vi "FeedbackDecode_BuildMSMSMvnt.vi"(4 "CompArray":T2(array[cluster])=[{"Name"="\"LittleSphereJ\"", "Type"="\"Trans3Joint\"", "ID"="J", "Num"="86", "COM"=[], "Offset"=[], "RotationAxis"=[], "OrientationMatrix"=[[1.0, 0.0, 0.0], [0.0, 1.0, 0.0], [0.0, 0.0, 1.0]], "MinAngle"=nan, "MaxAngle"=nan, "InboardID"="S", "InboardNum"="1110", "InboardCOM"=[0.0, 0.0, 0.0], "OutboardID"="S", "OutboardNum"="84", "OutboardCOM"=[0.0, 0.0, 0.0]}, {"Name"="\"IndexSphereJ\"", "Type"="\"Trans3Joint\"", "ID"="J", "Num"="94", "COM"=[], "Offset"=[], "RotationAxis"=[], "OrientationMatrix"=[[1.0, 0.0, 0.0], [0.0, 1.0, 0.0], [0.0, 0.0, 1.0]], "MinAngle"=nan, "MaxAngle"=nan, "InboardID"="S", "InboardNum"="1110", "InboardCOM"=[0.0, 0.0, 0.0], "OutboardID"="S", "OutboardNum"="92", "OutboardCOM"=[0.0, 0.0, 0.0]}, {"Name"="\"LittleKnuckle\"", "Type"="\"PinJoint\"", "ID"="J", "Num"="1160", "COM"=[], "Offset"=[], "RotationAxis"=[-0.982409, 0.0686967, 0.173648], "OrientationMatrix"=[[1.0, 0.0, 0.0], [0.0, 1.0, 0.0], [0.0, 0.0, 1.0]], "MinAngle"=0.0, "MaxAngle"=3.140021857262998, "InboardID"="S", "InboardNum"="1122", "InboardCOM"=[-0.01026417, -0.01431899999999997, 0.005183300000000002], "OutboardID"="S", "OutboardNum"="112", "OutboardCOM"=[0.0, 0.0, 0.0]}, {"Name"="\"LittleSide\"", "Type"="\"PinJoint\"", "ID"="J", "Num"="1161", "COM"=[], "Offset"=[], "RotationAxis"=[0.173225, -0.0121131, -0.984808], "OrientationMatrix"=[[1.0, 0.0, 0.0], [0.0, 1.0, 0.0], [0.0, 0.0, 1.0]], "MinAngle"=0.0, "MaxAngle"=3.140021857262998, "InboardID"="S", "InboardNum"="1110", "InboardCOM"=[-0.02813713, -0.080592, -0.0049779], "OutboardID"="S", "OutboardNum"="1122", "OutboardCOM"=[0.0, 0.0, 0.0]}, {"Name"="\"RingPIP\"", "Type"="\"PinJoint\"", "ID"="J", "Num"="1162", "COM"=[], "Offset"=[], "RotationAxis"=[-0.993768, 0.069491, 0.0871557], "OrientationMatrix"=[[1.0, 0.0, 0.0], [0.0, 1.0, 0.0], [0.0, 0.0, 1.0]], "MinAngle"=0.0, "MaxAngle"=3.140021857262998, "InboardID"="S", "InboardNum"="1125", "InboardCOM"=[-0.00263497, -0.03339700000000001, 2.619999999999706e-05], "OutboardID"="S", "OutboardNum"="1121", "OutboardCOM"=[0.0, 0.0, 0.0]}, {"Name"="\"ThumbKnuckle\"", "Type"="\"PinJoint\"", "ID"="J", "Num"="1163", "COM"=[], "Offset"=[], "RotationAxis"=[-0.130028, -0.197163, -0.97171], "OrientationMatrix"=[[1.0, 0.0, 0.0], [0.0, 1.0, 0.0], [0.0, 0.0, 1.0]], "MinAngle"=0.0, "MaxAngle"=3.140021857262998, "InboardID"="S", "InboardNum"="1113", "InboardCOM"=[0.0221366, -0.0038129999999999553, 0.00214783], "OutboardID"="S", "OutboardNum"="111", "OutboardCOM"=[0.0, 0.0, 0.0]}, {"Name"="\"RingSide\"", "Type"="\"PinJoint\"", "ID"="J", "Num"="1164", "COM"=[], "Offset"=[], "RotationAxis"=[0.0869434, -0.00607968, -0.996195], "OrientationMatrix"=[[1.0, 0.0, 0.0], [0.0, 1.0, 0.0], [0.0, 0.0, 1.0]], "MinAngle"=0.0, "MaxAngle"=3.140021857262998, "InboardID"="S", "InboardNum"="1110", "InboardCOM"=[-0.0087988, -0.08356699999999995, -0.008058199999999998], "OutboardID"="S", "OutboardNum"="1123", "OutboardCOM"=[0.0, 0.0, 0.0]}, {"Name"="\"RingKnuckle\"", "Type"="\"PinJoint\"", "ID"="J", "Num"="1165", "COM"=[], "Offset"=[], "RotationAxis"=[-0.993768, 0.069491, 0.0871557], "OrientationMatrix"=[[1.0, 0.0, 0.0], [0.0, 1.0, 0.0], [0.0, 0.0, 1.0]], "MinAngle"=0.0, "MaxAngle"=3.140021857262998, "InboardID"="S", "InboardNum"="1123", "InboardCOM"=[-0.01067969, -0.014290000000000025, 0.0043582], "OutboardID"="S", "OutboardNum"="1125", "OutboardCOM"=[0.0, 0.0, 0.0]}, {"Name"="\"ShoulderRoll\"", "Type"="\"PinJoint\"", "ID"="J", "Num"="1166", "COM"=[], "Offset"=[], "RotationAxis"=[0.0, -1.0, 0.0], "OrientationMatrix"=[[1.0, 0.0, 0.0], [0.0, 1.0, 0.0], [0.0, 0.0, 1.0]], "MinAngle"=0.0, "MaxAngle"=3.140021857262998, "InboardID"="S", "InboardNum"="1127", "InboardCOM"=[0.0346, -0.26093099999999997, 0.0], "OutboardID"="S", "OutboardNum"="116", "OutboardCOM"=[0.0, 0.0, 0.0]}, {"Name"="\"MiddleDIP\"", "Type"="\"PinJoint\"", "ID"="J", "Num"="1167", "COM"=[], "Offset"=[], "RotationAxis"=[-1.0, 0.0, 0.0], "OrientationMatrix"=[[1.0, 0.0, 0.0], [0.0, 1.0, 0.0], [0.0, 0.0, 1.0]], "MinAngle"=0.0, "MaxAngle"=3.14, "InboardID"="S", "InboardNum"="113", "InboardCOM"=[0.0197, -0.022077000000000013, -0.0010000000000000009], "OutboardID"="S", "OutboardNum"="1114", "OutboardCOM"=[0.0, 0.0, 0.0]}, {"Name"="\"IndexDIP\"", "Type"="\"PinJoint\"", "ID"="J", "Num"="1168", "COM"=[], "Offset"=[], "RotationAxis"=[-1.0, 0.0, 0.0], "OrientationMatrix"=[[1.0, 0.0, 0.0], [0.0, 1.0, 0.0], [0.0, 0.0, 1.0]], "MinAngle"=0.0, "MaxAngle"=3.140021857262998, "InboardID"="S", "InboardNum"="1124", "InboardCOM"=[0.019699999999999995, -0.017971999999999988, -0.0009999999999999974], "OutboardID"="S", "OutboardNum"="1117", "OutboardCOM"=[0.0, 0.0, 0.0]}, {"Name"="\"IndexKnuckle\"", "Type"="\"PinJoint\"", "ID"="J", "Num"="1169", "COM"=[], "Offset"=[], "RotationAxis"=[-1.0, 0.0, 0.0], "OrientationMatrix"=[[1.0, 0.0, 0.0], [0.0, 1.0, 0.0], [0.0, 0.0, 1.0]], "MinAngle"=0.0, "MaxAngle"=3.140021857262998, "InboardID"="S", "InboardNum"="1118", "InboardCOM"=[-0.0071716, -0.017827999999999955, 0.0025407999999999993], "OutboardID"="S", "OutboardNum"="1126", "OutboardCOM"=[0.0, 0.0, 0.0]}, {"Name"="\"MiddleKnuckle\"", "Type"="\"PinJoint\"", "ID"="J", "Num"="1170", "COM"=[], "Offset"=[], "RotationAxis"=[-1.0, 0.0, 0.0], "OrientationMatrix"=[[1.0, 0.0, 0.0], [0.0, 1.0, 0.0], [0.0, 0.0, 1.0]], "MinAngle"=0.0, "MaxAngle"=3.140021857262998, "InboardID"="S", "InboardNum"="1110", "InboardCOM"=[-0.00031180000000000097, -0.09855000000000003, -0.0048641], "OutboardID"="S", "OutboardNum"="1119", "OutboardCOM"=[0.0, 0.0, 0.0]}, {"Name"="\"RingSphereJ\"", "Type"="\"Trans3Joint\"", "ID"="J", "Num"="15", "COM"=[], "Offset"=[], "RotationAxis"=[], "OrientationMatrix"=[[1.0, 0.0, 0.0], [0.0, 1.0, 0.0], [0.0, 0.0, 1.0]], "MinAngle"=nan, "MaxAngle"=nan, "InboardID"="S", "InboardNum"="1110", "InboardCOM"=[0.0, 0.0, 0.0], "OutboardID"="S", "OutboardNum"="18", "OutboardCOM"=[0.0, 0.0, 0.0]}, {"Name"="\"MiddleSphereJ\"", "Type"="\"Trans3Joint\"", "ID"="J", "Num"="11", "COM"=[], "Offset"=[], "RotationAxis"=[], "OrientationMatrix"=[[1.0, 0.0, 0.0], [0.0, 1.0, 0.0], [0.0, 0.0, 1.0]], "MinAngle"=nan, "MaxAngle"=nan, "InboardID"="S", "InboardNum"="1110", "InboardCOM"=[0.0, 0.0, 0.0], "OutboardID"="S", "OutboardNum"="14", "OutboardCOM"=[0.0, 0.0, 0.0]}, {"Name"="\"ThumbSphereJ\"", "Type"="\"Trans3Joint\"", "ID"="J", "Num"="23", "COM"=[], "Offset"=[], "RotationAxis"=[], "OrientationMatrix"=[[1.0, 0.0, 0.0], [0.0, 1.0, 0.0], [0.0, 0.0, 1.0]], "MinAngle"=nan, "MaxAngle"=nan, "InboardID"="S", "InboardNum"="1110", "InboardCOM"=[0.0, 0.0, 0.0], "OutboardID"="S", "OutboardNum"="22", "OutboardCOM"=[0.0, 0.0, 0.0]}, {"Name"="\"RingDIP\"", "Type"="\"PinJoint\"", "ID"="J", "Num"="1144", "COM"=[], "Offset"=[], "RotationAxis"=[-0.993768, 0.069491, 0.0871557], "OrientationMatrix"=[[1.0, 0.0, 0.0], [0.0, 1.0, 0.0], [0.0, 0.0, 1.0]], "MinAngle"=0.0, "MaxAngle"=3.140021857262998, "InboardID"="S", "InboardNum"="1121", "InboardCOM"=[0.01818386, -0.020046000000000008, -0.002713199999999999], "OutboardID"="S", "OutboardNum"="115", "OutboardCOM"=[0.0, 0.0, 0.0]}, {"Name"="\"ElbowPitch\"", "Type"="\"PinJoint\"", "ID"="J", "Num"="1145", "COM"=[], "Offset"=[], "RotationAxis"=[0.0, 0.0, 1.0], "OrientationMatrix"=[[1.0, 0.0, 0.0], [0.0, 1.0, 0.0], [0.0, 0.0, 1.0]], "MinAngle"=0.0, "MaxAngle"=3.140021857262998, "InboardID"="S", "InboardNum"="116", "InboardCOM"=[0.019, -0.013836000000000015, -0.009000000000000001], "OutboardID"="S", "OutboardNum"="1111", "OutboardCOM"=[0.0, 0.0, 0.0]}, {"Name"="\"WristPitch\"", "Type"="\"PinJoint\"", "ID"="J", "Num"="1146", "COM"=[], "Offset"=[], "RotationAxis"=[-1.0, 0.0, 0.0], "OrientationMatrix"=[[1.0, 0.0, 0.0], [0.0, 1.0, 0.0], [0.0, 0.0, 1.0]], "MinAngle"=-0.7853981633974483, "MaxAngle"=0.7853981633974483, "InboardID"="S", "InboardNum"="114", "InboardCOM"=[0.042499999999999996, -0.16914000000000007, 0.0], "OutboardID"="S", "OutboardNum"="119", "OutboardCOM"=[0.0, 0.0, 0.0]}, {"Name"="\"ThumbDIP\"", "Type"="\"PinJoint\"", "ID"="J", "Num"="1147", "COM"=[], "Offset"=[], "RotationAxis"=[-0.130028, -0.197163, -0.97171], "OrientationMatrix"=[[1.0, 0.0, 0.0], [0.0, 1.0, 0.0], [0.0, 0.0, 1.0]], "MinAngle"=0.0, "MaxAngle"=3.14, "InboardID"="S", "InboardNum"="111", "InboardCOM"=[0.018637, -0.022448000000000023, -0.01061123], "OutboardID"="S", "OutboardNum"="1116", "OutboardCOM"=[0.0, 0.0, 0.0]}, {"Name"="\"IndexSide\"", "Type"="\"PinJoint\"", "ID"="J", "Num"="1148", "COM"=[], "Offset"=[], "RotationAxis"=[0.0, 0.0, -1.0], "OrientationMatrix"=[[1.0, 0.0, 0.0], [0.0, 1.0, 0.0], [0.0, 0.0, 1.0]], "MinAngle"=0.0, "MaxAngle"=3.140021857262998, "InboardID"="S", "InboardNum"="1110", "InboardCOM"=[0.027229700000000003, -0.07779400000000003, -0.0051141], "OutboardID"="S", "OutboardNum"="1118", "OutboardCOM"=[0.0, 0.0, 0.0]}, {"Name"="\"MiddlePIP\"", "Type"="\"PinJoint\"", "ID"="J", "Num"="1149", "COM"=[], "Offset"=[], "RotationAxis"=[-1.0, 0.0, 0.0], "OrientationMatrix"=[[1.0, 0.0, 0.0], [0.0, 1.0, 0.0], [0.0, 0.0, 1.0]], "MinAngle"=0.0, "MaxAngle"=3.140021857262998, "InboardID"="S", "InboardNum"="1119", "InboardCOM"=[-0.0002999999999999982, -0.0383, 0.0], "OutboardID"="S", "OutboardNum"="113", "OutboardCOM"=[0.0, 0.0, 0.0]}, {"Name"="\"ShoulderYaw\"", "Type"="\"PinJoint\"", "ID"="J", "Num"="1150", "COM"=[], "Offset"=[], "RotationAxis"=[0.0, 0.0, 1.0], "OrientationMatrix"=[[1.0, 0.0, 0.0], [0.0, 1.0, 0.0], [0.0, 0.0, 1.0]], "MinAngle"=0.0, "MaxAngle"=3.140021857262998, "InboardID"="S", "InboardNum"="117", "InboardCOM"=[-1.45121e-10, 0.000384746, -0.003098433], "OutboardID"="S", "OutboardNum"="1120", "OutboardCOM"=[0.0, 0.0, 0.0]}, {"Name"="\"ThumbSide\"", "Type"="\"PinJoint\"", "ID"="J", "Num"="1151", "COM"=[], "Offset"=[], "RotationAxis"=[0.691978, 0.683845, -0.23135], "OrientationMatrix"=[[1.0, 0.0, 0.0], [0.0, 1.0, 0.0], [0.0, 0.0, 1.0]], "MinAngle"=-0.7853981633974483, "MaxAngle"=0.7853981633974483, "InboardID"="S", "InboardNum"="118", "InboardCOM"=[0.008416800000000002, -0.028861000000000026, 0.0017169000000000004], "OutboardID"="S", "OutboardNum"="1113", "OutboardCOM"=[0.0, 0.0, 0.0]}, {"Name"="\"LittleDIP\"", "Type"="\"PinJoint\"", "ID"="J", "Num"="1152", "COM"=[], "Offset"=[], "RotationAxis"=[-0.982409, 0.0686967, 0.173648], "OrientationMatrix"=[[1.0, 0.0, 0.0], [0.0, 1.0, 0.0], [0.0, 0.0, 1.0]], "MinAngle"=0.0, "MaxAngle"=3.140021857262998, "InboardID"="S", "InboardNum"="1115", "InboardCOM"=[0.01887955, -0.014112000000000013, -0.004509900000000001], "OutboardID"="S", "OutboardNum"="1112", "OutboardCOM"=[0.0, 0.0, 0.0]}, {"Name"="\"WristYaw\"", "Type"="\"PinJoint\"", "ID"="J", "Num"="1153", "COM"=[], "Offset"=[], "RotationAxis"=[0.0, 0.0, -1.0], "OrientationMatrix"=[[1.0, 0.0, 0.0], [0.0, 1.0, 0.0], [0.0, 0.0, 1.0]], "MinAngle"=-0.7853981633974483, "MaxAngle"=0.7853981633974483, "InboardID"="S", "InboardNum"="119", "InboardCOM"=[-0.0425218, -0.006901999999999964, -0.004796100000000001], "OutboardID"="S", "OutboardNum"="1110", "OutboardCOM"=[0.0, 0.0, 0.0]}, {"Name"="\"IndexPIP\"", "Type"="\"PinJoint\"", "ID"="J", "Num"="1154", "COM"=[], "Offset"=[], "RotationAxis"=[-1.0, 0.0, 0.0], "OrientationMatrix"=[[1.0, 0.0, 0.0], [0.0, 1.0, 0.0], [0.0, 0.0, 1.0]], "MinAngle"=0.0, "MaxAngle"=3.140021857262998, "InboardID"="S", "InboardNum"="1126", "InboardCOM"=[-0.00030000000000000165, -0.03400000000000003, 0.0], "OutboardID"="S", "OutboardNum"="1124", "OutboardCOM"=[0.0, 0.0, 0.0]}, {"Name"="\"LittlePIP\"", "Type"="\"PinJoint\"", "ID"="J", "Num"="1155", "COM"=[], "Offset"=[], "RotationAxis"=[-0.982409, 0.0686967, 0.173648], "OrientationMatrix"=[[1.0, 0.0, 0.0], [0.0, 1.0, 0.0], [0.0, 0.0, 1.0]], "MinAngle"=0.0, "MaxAngle"=3.140021857262998, "InboardID"="S", "InboardNum"="112", "InboardCOM"=[-0.0021084, -0.02591600000000005, 5.209999999999937e-05], "OutboardID"="S", "OutboardNum"="1115", "OutboardCOM"=[0.0, 0.0, 0.0]}, {"Name"="\"ThumbMeta\"", "Type"="\"PinJoint\"", "ID"="J", "Num"="1156", "COM"=[], "Offset"=[], "RotationAxis"=[-0.0212682, -0.997909, -0.0610298], "OrientationMatrix"=[[1.0, 0.0, 0.0], [0.0, 1.0, 0.0], [0.0, 0.0, 1.0]], "MinAngle"=0.0, "MaxAngle"=3.14, "InboardID"="S", "InboardNum"="1110", "InboardCOM"=[0.015011799999999999, -0.011859999999999982, 0.0126182], "OutboardID"="S", "OutboardNum"="118", "OutboardCOM"=[0.0, 0.0, 0.0]}, {"Name"="\"ShoulderOblique\"", "Type"="\"PinJoint\"", "ID"="J", "Num"="1157", "COM"=[], "Offset"=[], "RotationAxis"=[0.57735, 0.57735, 0.57735], "OrientationMatrix"=[[1.0, 0.0, 0.0], [0.0, 1.0, 0.0], [0.0, 0.0, 1.0]], "MinAngle"=0.0, "MaxAngle"=3.14, "InboardID"="S", "InboardNum"="12", "InboardCOM"=[-0.09, -0.05, -0.26], "OutboardID"="S", "OutboardNum"="117", "OutboardCOM"=[0.0, 0.0, 0.0]}, {"Name"="\"ShoulderPitch\"", "Type"="\"PinJoint\"", "ID"="J", "Num"="1158", "COM"=[], "Offset"=[], "RotationAxis"=[-1.0, 0.0, 0.0], "OrientationMatrix"=[[1.0, 0.0, 0.0], [0.0, 1.0, 0.0], [0.0, 0.0, 1.0]], "MinAngle"=0.0, "MaxAngle"=3.140021857262998, "InboardID"="S", "InboardNum"="1120", "InboardCOM"=[-0.0346, -0.005, -0.0125], "OutboardID"="S", "OutboardNum"="1127", "OutboardCOM"=[0.0, 0.0, 0.0]}, {"Name"="\"WristRoll\"", "Type"="\"PinJoint\"", "ID"="J", "Num"="1159", "COM"=[], "Offset"=[], "RotationAxis"=[0.0, -1.0, 0.0], "OrientationMatrix"=[[1.0, 0.0, 0.0], [0.0, 1.0, 0.0], [0.0, 0.0, 1.0]], "MinAngle"=-1.5707963267948966, "MaxAngle"=1.5707963267948966, "InboardID"="S", "InboardNum"="1111", "InboardCOM"=[0.0, -0.06298999999999999, 0.003020000000000002], "OutboardID"="S", "OutboardNum"="114", "OutboardCOM"=[0.0, 0.0, 0.0]}, {"Name"="\"WristSphereJ\"", "Type"="\"Trans3Joint\"", "ID"="J", "Num"="88", "COM"=[], "Offset"=[], "RotationAxis"=[], "OrientationMatrix"=[[1.0, 0.0, 0.0], [0.0, 1.0, 0.0], [0.0, 0.0, 1.0]], "MinAngle"=nan, "MaxAngle"=nan, "InboardID"="S", "InboardNum"="114", "InboardCOM"=[0.0, 0.0, 0.0], "OutboardID"="S", "OutboardNum"="87", "OutboardCOM"=[0.0, 0.0, 0.0]}, {"Name"="\"LittleSphere\"", "Type"="\"Segment\"", "ID"="S", "Num"="84", "COM"=[0.0, 0.0, 0.0], "Offset"=[0.0, 0.0, 0.0], "RotationAxis"=[], "OrientationMatrix"=[], "MinAngle"=nan, "MaxAngle"=nan, "InboardID"="", "InboardNum"="", "InboardCOM"=[], "OutboardID"="", "OutboardNum"="", "OutboardCOM"=[]}, {"Name"="\"IndexSphere\"", "Type"="\"Segment\"", "ID"="S", "Num"="92", "COM"=[0.0, 0.0, 0.0], "Offset"=[0.0, 0.0, 0.0], "RotationAxis"=[], "OrientationMatrix"=[], "MinAngle"=nan, "MaxAngle"=nan, "InboardID"="", "InboardNum"="", "InboardCOM"=[], "OutboardID"="", "OutboardNum"="", "OutboardCOM"=[]}, {"Name"="\"ShoulderHR\"", "Type"="\"Segment\"", "ID"="S", "Num"="1127", "COM"=[0.03942751, -0.096221, -2.3999999999996247e-06], "Offset"=[0.0346, 0.005, 0.01541], "RotationAxis"=[], "OrientationMatrix"=[], "MinAngle"=nan, "MaxAngle"=nan, "InboardID"="", "InboardNum"="", "InboardCOM"=[], "OutboardID"="", "OutboardNum"="", "OutboardCOM"=[]}, {"Name"="\"ThumbProximal\"", "Type"="\"Segment\"", "ID"="S", "Num"="111", "COM"=[0.010053400000000004, -0.01129800000000003, -0.003517029999999999], "Offset"=[-0.0645434, 0.563333, 0.00970317], "RotationAxis"=[], "OrientationMatrix"=[], "MinAngle"=nan, "MaxAngle"=nan, "InboardID"="", "InboardNum"="", "InboardCOM"=[], "OutboardID"="", "OutboardNum"="", "OutboardCOM"=[]}, {"Name"="\"LittleProximal\"", "Type"="\"Segment\"", "ID"="S", "Num"="112", "COM"=[0.0086144, -0.013174000000000019, -0.0019825000000000016], "Offset"=[0.0194231, 0.61371, 0.0259807], "RotationAxis"=[], "OrientationMatrix"=[], "MinAngle"=nan, "MaxAngle"=nan, "InboardID"="", "InboardNum"="", "InboardCOM"=[], "OutboardID"="", "OutboardNum"="", "OutboardCOM"=[]}, {"Name"="\"MiddleMedial\"", "Type"="\"Segment\"", "ID"="S", "Num"="113", "COM"=[0.009050299999999997, -0.011116000000000015, -0.0009771999999999975], "Offset"=[-0.0183664, 0.655649, 0.0310502], "RotationAxis"=[], "OrientationMatrix"=[], "MinAngle"=nan, "MaxAngle"=nan, "InboardID"="", "InboardNum"="", "InboardCOM"=[], "OutboardID"="", "OutboardNum"="", "OutboardCOM"=[]}, {"Name"="\"Forearm\"", "Type"="\"Segment\"", "ID"="S", "Num"="114", "COM"=[-1.860000000000056e-05, -0.08232500000000004, -9.750000000000036e-05], "Offset"=[-0.019, 0.342757, 0.02139], "RotationAxis"=[], "OrientationMatrix"=[], "MinAngle"=nan, "MaxAngle"=nan, "InboardID"="", "InboardNum"="", "InboardCOM"=[], "OutboardID"="", "OutboardNum"="", "OutboardCOM"=[]}, {"Name"="\"RingDistal\"", "Type"="\"Segment\"", "ID"="S", "Num"="115", "COM"=[-0.01039068, -0.008301000000000003, 0.0005073999999999981], "Offset"=[-0.0150486, 0.670099, 0.0325731], "RotationAxis"=[], "OrientationMatrix"=[], "MinAngle"=nan, "MaxAngle"=nan, "InboardID"="", "InboardNum"="", "InboardCOM"=[], "OutboardID"="", "OutboardNum"="", "OutboardCOM"=[]}, {"Name"="\"HR TO ELBOW_1\"", "Type"="\"Segment\"", "ID"="S", "Num"="116", "COM"=[0.0103972, 0.026906999999999986, 0.0011380000000000001], "Offset"=[0.0, 0.265931, 0.01541], "RotationAxis"=[], "OrientationMatrix"=[], "MinAngle"=nan, "MaxAngle"=nan, "InboardID"="", "InboardNum"="", "InboardCOM"=[], "OutboardID"="", "OutboardNum"="", "OutboardCOM"=[]}, {"Name"="\"ShoulderSocket\"", "Type"="\"Segment\"", "ID"="S", "Num"="117", "COM"=[0.0, 0.0, 0.0], "Offset"=[-1.45121e-10, 0.000384746, -0.000188433], "RotationAxis"=[], "OrientationMatrix"=[], "MinAngle"=nan, "MaxAngle"=nan, "InboardID"="", "InboardNum"="", "InboardCOM"=[], "OutboardID"="", "OutboardNum"="", "OutboardCOM"=[]}, {"Name"="\"ThumbRoll\"", "Type"="\"Segment\"", "ID"="S", "Num"="118", "COM"=[0.005574799999999998, -0.01721499999999998, -0.0012329999999999997], "Offset"=[-0.03399, 0.530659, 0.0135679], "RotationAxis"=[], "OrientationMatrix"=[], "MinAngle"=nan, "MaxAngle"=nan, "InboardID"="", "InboardNum"="", "InboardCOM"=[], "OutboardID"="", "OutboardNum"="", "OutboardCOM"=[]}, {"Name"="\"WristFlex\"", "Type"="\"Segment\"", "ID"="S", "Num"="119", "COM"=[-0.0420033, -0.003865999999999925, 0.000690699999999999], "Offset"=[-0.0615, 0.511897, 0.02139], "RotationAxis"=[], "OrientationMatrix"=[], "MinAngle"=nan, "MaxAngle"=nan, "InboardID"="", "InboardNum"="", "InboardCOM"=[], "OutboardID"="", "OutboardNum"="", "OutboardCOM"=[]}, {"Name"="\"ThumbSphere\"", "Type"="\"Segment\"", "ID"="S", "Num"="22", "COM"=[0.0, 0.0, 0.0], "Offset"=[0.0, 0.0, 0.0], "RotationAxis"=[], "OrientationMatrix"=[], "MinAngle"=nan, "MaxAngle"=nan, "InboardID"="", "InboardNum"="", "InboardCOM"=[], "OutboardID"="", "OutboardNum"="", "OutboardCOM"=[]}, {"Name"="\"RingSphere\"", "Type"="\"Segment\"", "ID"="S", "Num"="18", "COM"=[0.0, 0.0, 0.0], "Offset"=[0.0, 0.0, 0.0], "RotationAxis"=[], "OrientationMatrix"=[], "MinAngle"=nan, "MaxAngle"=nan, "InboardID"="", "InboardNum"="", "InboardCOM"=[], "OutboardID"="", "OutboardNum"="", "OutboardCOM"=[]}, {"Name"="\"MiddleSphere\"", "Type"="\"Segment\"", "ID"="S", "Num"="14", "COM"=[0.0, 0.0, 0.0], "Offset"=[0.0, 0.0, 0.0], "RotationAxis"=[], "OrientationMatrix"=[], "MinAngle"=nan, "MaxAngle"=nan, "InboardID"="", "InboardNum"="", "InboardCOM"=[], "OutboardID"="", "OutboardNum"="", "OutboardCOM"=[]}, {"Name"="\"PalmAssembly\"", "Type"="\"Segment\"", "ID"="S", "Num"="1110", "COM"=[5.000000000005e-07, -0.049819999999999975, 0.0028357999999999994], "Offset"=[-0.0189782, 0.518799, 0.0261861], "RotationAxis"=[], "OrientationMatrix"=[], "MinAngle"=nan, "MaxAngle"=nan, "InboardID"="", "InboardNum"="", "InboardCOM"=[], "OutboardID"="", "OutboardNum"="", "OutboardCOM"=[]}, {"Name"="\"ELBOW TO RR_1\"", "Type"="\"Segment\"", "ID"="S", "Num"="1111", "COM"=[-0.0009622999999999993, -0.06578500000000004, 0.0023389000000000014], "Offset"=[-0.019, 0.279767, 0.02441], "RotationAxis"=[], "OrientationMatrix"=[], "MinAngle"=nan, "MaxAngle"=nan, "InboardID"="", "InboardNum"="", "InboardCOM"=[], "OutboardID"="", "OutboardNum"="", "OutboardCOM"=[]}, {"Name"="\"LittleDistal\"", "Type"="\"Segment\"", "ID"="S", "Num"="1112", "COM"=[-0.01022215, -0.006736999999999993, 0.0015411999999999995], "Offset"=[0.00265195, 0.653738, 0.0304385], "RotationAxis"=[], "OrientationMatrix"=[], "MinAngle"=nan, "MaxAngle"=nan, "InboardID"="", "InboardNum"="", "InboardCOM"=[], "OutboardID"="", "OutboardNum"="", "OutboardCOM"=[]}, {"Name"="\"ThumbMedial\"", "Type"="\"Segment\"", "ID"="S", "Num"="1113", "COM"=[0.014731999999999995, 0.003503000000000034, -0.0037245000000000004], "Offset"=[-0.0424068, 0.55952, 0.011851], "RotationAxis"=[], "OrientationMatrix"=[], "MinAngle"=nan, "MaxAngle"=nan, "InboardID"="", "InboardNum"="", "InboardCOM"=[], "OutboardID"="", "OutboardNum"="", "OutboardCOM"=[]}, {"Name"="\"MiddleDistal\"", "Type"="\"Segment\"", "ID"="S", "Num"="1114", "COM"=[-0.0100904, -0.008909999999999973, -0.00043409999999999976], "Offset"=[-0.0380664, 0.677726, 0.0320502], "RotationAxis"=[], "OrientationMatrix"=[], "MinAngle"=nan, "MaxAngle"=nan, "InboardID"="", "InboardNum"="", "InboardCOM"=[], "OutboardID"="", "OutboardNum"="", "OutboardCOM"=[]}, {"Name"="\"LittleMedial\"", "Type"="\"Segment\"", "ID"="S", "Num"="1115", "COM"=[0.009976699999999998, -0.005878999999999968, -0.002634000000000001], "Offset"=[0.0215315, 0.639626, 0.0259286], "RotationAxis"=[], "OrientationMatrix"=[], "MinAngle"=nan, "MaxAngle"=nan, "InboardID"="", "InboardNum"="", "InboardCOM"=[], "OutboardID"="", "OutboardNum"="", "OutboardCOM"=[]}, {"Name"="\"ThumbDistal\"", "Type"="\"Segment\"", "ID"="S", "Num"="1116", "COM"=[0.0094852, -0.005989000000000022, 0.008354], "Offset"=[-0.0831804, 0.585781, 0.0203144], "RotationAxis"=[], "OrientationMatrix"=[], "MinAngle"=nan, "MaxAngle"=nan, "InboardID"="", "InboardNum"="", "InboardCOM"=[], "OutboardID"="", "OutboardNum"="", "OutboardCOM"=[]}, {"Name"="\"IndexDistal\"", "Type"="\"Segment\"", "ID"="S", "Num"="1117", "COM"=[-0.009959199999999994, -0.007608999999999977, -6.570000000000187e-05], "Offset"=[-0.0584363, 0.666393, 0.0297594], "RotationAxis"=[], "OrientationMatrix"=[], "MinAngle"=nan, "MaxAngle"=nan, "InboardID"="", "InboardNum"="", "InboardCOM"=[], "OutboardID"="", "OutboardNum"="", "OutboardCOM"=[]}, {"Name"="\"MCPIndex\"", "Type"="\"Segment\"", "ID"="S", "Num"="1118", "COM"=[0.0017073999999999978, -0.006472999999999951, 0.002308899999999999], "Offset"=[-0.0462079, 0.596593, 0.0313002], "RotationAxis"=[], "OrientationMatrix"=[], "MinAngle"=nan, "MaxAngle"=nan, "InboardID"="", "InboardNum"="", "InboardCOM"=[], "OutboardID"="", "OutboardNum"="", "OutboardCOM"=[]}, {"Name"="\"MiddleProximal\"", "Type"="\"Segment\"", "ID"="S", "Num"="1119", "COM"=[0.009659500000000001, -0.017927999999999944, -8.019999999999902e-05], "Offset"=[-0.0186664, 0.617349, 0.0310502], "RotationAxis"=[], "OrientationMatrix"=[], "MinAngle"=nan, "MaxAngle"=nan, "InboardID"="", "InboardNum"="", "InboardCOM"=[], "OutboardID"="", "OutboardNum"="", "OutboardCOM"=[]}, {"Name"="\"ShoulderGearMotor\"", "Type"="\"Segment\"", "ID"="S", "Num"="1120", "COM"=[0.0067537, -0.00104092, -0.0093986], "Offset"=[0.0, 0.0, 0.00291], "RotationAxis"=[], "OrientationMatrix"=[], "MinAngle"=nan, "MaxAngle"=nan, "InboardID"="", "InboardNum"="", "InboardCOM"=[], "OutboardID"="", "OutboardNum"="", "OutboardCOM"=[]}, {"Name"="\"RingMedial\"", "Type"="\"Segment\"", "ID"="S", "Num"="1121", "COM"=[0.00875476, -0.00992700000000002, -0.0017671999999999966], "Offset"=[0.00313526, 0.650053, 0.0298599], "RotationAxis"=[], "OrientationMatrix"=[], "MinAngle"=nan, "MaxAngle"=nan, "InboardID"="", "InboardNum"="", "InboardCOM"=[], "OutboardID"="", "OutboardNum"="", "OutboardCOM"=[]}, {"Name"="\"MCPLittle\"", "Type"="\"Segment\"", "ID"="S", "Num"="1122", "COM"=[4.4959999999998404e-05, -0.007433999999999941, 0.0037990000000000003], "Offset"=[0.00915893, 0.599391, 0.031164], "RotationAxis"=[], "OrientationMatrix"=[], "MinAngle"=nan, "MaxAngle"=nan, "InboardID"="", "InboardNum"="", "InboardCOM"=[], "OutboardID"="", "OutboardNum"="", "OutboardCOM"=[]}, {"Name"="\"MCPRing\"", "Type"="\"Segment\"", "ID"="S", "Num"="1123", "COM"=[0.00014349999999999953, -0.007109000000000032, 0.003743], "Offset"=[-0.0101794, 0.602366, 0.0342443], "RotationAxis"=[], "OrientationMatrix"=[], "MinAngle"=nan, "MaxAngle"=nan, "InboardID"="", "InboardNum"="", "InboardCOM"=[], "OutboardID"="", "OutboardNum"="", "OutboardCOM"=[]}, {"Name"="\"IndexMedial\"", "Type"="\"Segment\"", "ID"="S", "Num"="1124", "COM"=[0.009597399999999999, -0.008967999999999976, -0.0012315999999999994], "Offset"=[-0.0387363, 0.648421, 0.0287594], "RotationAxis"=[], "OrientationMatrix"=[], "MinAngle"=nan, "MaxAngle"=nan, "InboardID"="", "InboardNum"="", "InboardCOM"=[], "OutboardID"="", "OutboardNum"="", "OutboardCOM"=[]}, {"Name"="\"RingProximal\"", "Type"="\"Segment\"", "ID"="S", "Num"="1125", "COM"=[0.008387790000000001, -0.01778599999999997, -0.0011962000000000014], "Offset"=[0.00050029, 0.616656, 0.0298861], "RotationAxis"=[], "OrientationMatrix"=[], "MinAngle"=nan, "MaxAngle"=nan, "InboardID"="", "InboardNum"="", "InboardCOM"=[], "OutboardID"="", "OutboardNum"="", "OutboardCOM"=[]}, {"Name"="\"IndexProximal\"", "Type"="\"Segment\"", "ID"="S", "Num"="1126", "COM"=[0.010082999999999995, -0.01634599999999997, -0.00038749999999999896], "Offset"=[-0.0390363, 0.614421, 0.0287594], "RotationAxis"=[], "OrientationMatrix"=[], "MinAngle"=nan, "MaxAngle"=nan, "InboardID"="", "InboardNum"="", "InboardCOM"=[], "OutboardID"="", "OutboardNum"="", "OutboardCOM"=[]}, {"Name"="\"WristSphere\"", "Type"="\"Segment\"", "ID"="S", "Num"="87", "COM"=[0.0, 0.0, 0.0], "Offset"=[0.0, 0.0, 0.0], "RotationAxis"=[], "OrientationMatrix"=[], "MinAngle"=nan, "MaxAngle"=nan, "InboardID"="", "InboardNum"="", "InboardCOM"=[], "OutboardID"="", "OutboardNum"="", "OutboardCOM"=[]}], 6 "ModelParams":T1, 7 "MvntArray":dbl[](array[numeric])=[0.0, 0.0, 0.0, 0.0, 0.0, 0.0, 0.0, 0.0, 0.0, 0.0, 0.0, 0.0] min=-1.0 max=1.0, 9 "Mode":enum16{"Initialize", "Run"}(ring)) -> (0 "CompVals":sgl[][](array[numeric])=[[0.3926991], [0.43633232], [0.65449846], [0.65449846], [0.65449846], [0.3926991], [0.65449846], [0.65449846], [0.3926991], [0.65449846], [0.65449846], [0.3926991], [0.65449846], [0.65449846], [0.3926991], [0.0], [-0.02617994], [0.0], [0.061086524]], 1 "FNums":i16[](array[numeric])=[1, 1, 1, 1, 1, 1, 1, 1, 1, 1, 1, 1, 1, 1, 1, 1, 1, 1, 1], 3 "CompIdxs":i32[](array[numeric])=[28, 5, 19, 11, 26, 10, 12, 21, 9, 7, 4, 16, 2, 27, 24, 23, 20, 6, 3])   [LabVIEW 2020]
uses:
  C:/Users/Administrator/Documents/LabVIEW Data/MathScriptVIs/MCStatic_53690370032_474a7dcd89ebe4926e43c698fd5ec01d.vi
  <instcachedir>/0/MCStatic_53690370032_474a7dcd89ebe4926e43c698fd5ec01d_959F8FE6B6AA4F168807C51B34C1D6E7.lvgen/MCStatic_53690370032_474a7dcd89ebe4926e43c698fd5ec01d_959F8FE6B6AA4F168807C51B34C1D6E7_002.vi
  <vilib>/imath/engines/lvmath2/RunTimeEngine/NodeEndStatement/NIMS_NodeEndStatement_Output.vi
  <instcachedir>/0/NIMS_NodeEndStatement_Output_53EC0D466D134D7ABD903AC30B43404B.lvgen/NIMS_NodeEndStatement_Output_53EC0D466D134D7ABD903AC30B43404B_005.vi
  <vilib>/imath/engines/lvmath2/RunTimeEngine/ErrorHandling/NIMS_Finalize Error.vi
  FeedbackDecode_interpCompBnds.m
panel:
  in  "MvntCluster":T3(array[cluster])=[{"Name"="Thumb", "CompNames"=["\"ThumbMeta\"", "\"ThumbKnuckle\"", "\"ThumbDIP\""], "FNums"=[1, 1, 1], "CompIdxs"=[28, 5, 19], "CompBnds"=[[0.0, 45.0], [0.0, 50.0], [0.0, 75.0]]}, {"Name"="Index", "CompNames"=["\"IndexKnuckle\"", "\"IndexPIP\"", "\"IndexDIP\""], "FNums"=[1, 1, 1], "CompIdxs"=[11, 26, 10], "CompBnds"=[[0.0, 75.0], [0.0, 75.0], [0.0, 45.0]]}, {"Name"="Middle\n", "CompNames"=["\"MiddleKnuckle\"", "\"MiddlePIP\"", "\"MiddleDIP\""], "FNums"=[1, 1, 1], "CompIdxs"=[12, 21, 9], "CompBnds"=[[0.0, 75.0], [0.0, 75.0], [0.0, 45.0]]}, {"Name"="Ring", "CompNames"=["\"RingKnuckle\"", "\"RingPIP\"", "\"RingDIP\""], "FNums"=[1, 1, 1], "CompIdxs"=[7, 4, 16], "CompBnds"=[[0.0, 75.0], [0.0, 75.0], [0.0, 45.0]]}, {"Name"="Little", "CompNames"=["\"LittleKnuckle\"", "\"LittlePIP\"", "\"LittleDIP\""], "FNums"=[1, 1, 1], "CompIdxs"=[2, 27, 24], "CompBnds"=[[0.0, 75.0], [0.0, 75.0], [0.0, 45.0]]}, {"Name"="ThumbInt", "CompNames"=["\"ThumbSide\""], "FNums"=[1], "CompIdxs"=[23], "CompBnds"=[[-40.0, 40.0]]}, {"Name"="IndexInt", "CompNames"=["\"IndexSide\""], "FNums"=[1], "CompIdxs"=[20], "CompBnds"=[[10.0, -13.0]]}, {"Name"="RingInt", "CompNames"=["\"RingSide\""], "FNums"=[1], "CompIdxs"=[6], "CompBnds"=[[-10.0, 10.0]]}, {"Name"="LittleInt", "CompNames"=["\"LittleSide\""], "FNums"=[1], "CompIdxs"=[3], "CompBnds"=[[-8.0, 15.0]]}, {"Name"="WristPitch", "CompNames"=["\"WristPitch\""], "FNums"=[1], "CompIdxs"=[18], "CompBnds"=[[-45.0, 45.0]]}, {"Name"="WristYaw", "CompNames"=["\"WristYaw\""], "FNums"=[1], "CompIdxs"=[25], "CompBnds"=[[45.0, -45.0]]}, {"Name"="WristRoll", "CompNames"=["\"WristRoll\""], "FNums"=[1], "CompIdxs"=[], "CompBnds"=[]}]
  # "Thumb\nIndex\nMiddle\nRing\nLittle\nThumbInt\nIndexInt\nRingInt\nLittleInt\nWristPitch\nWristYaw\nWristRoll"
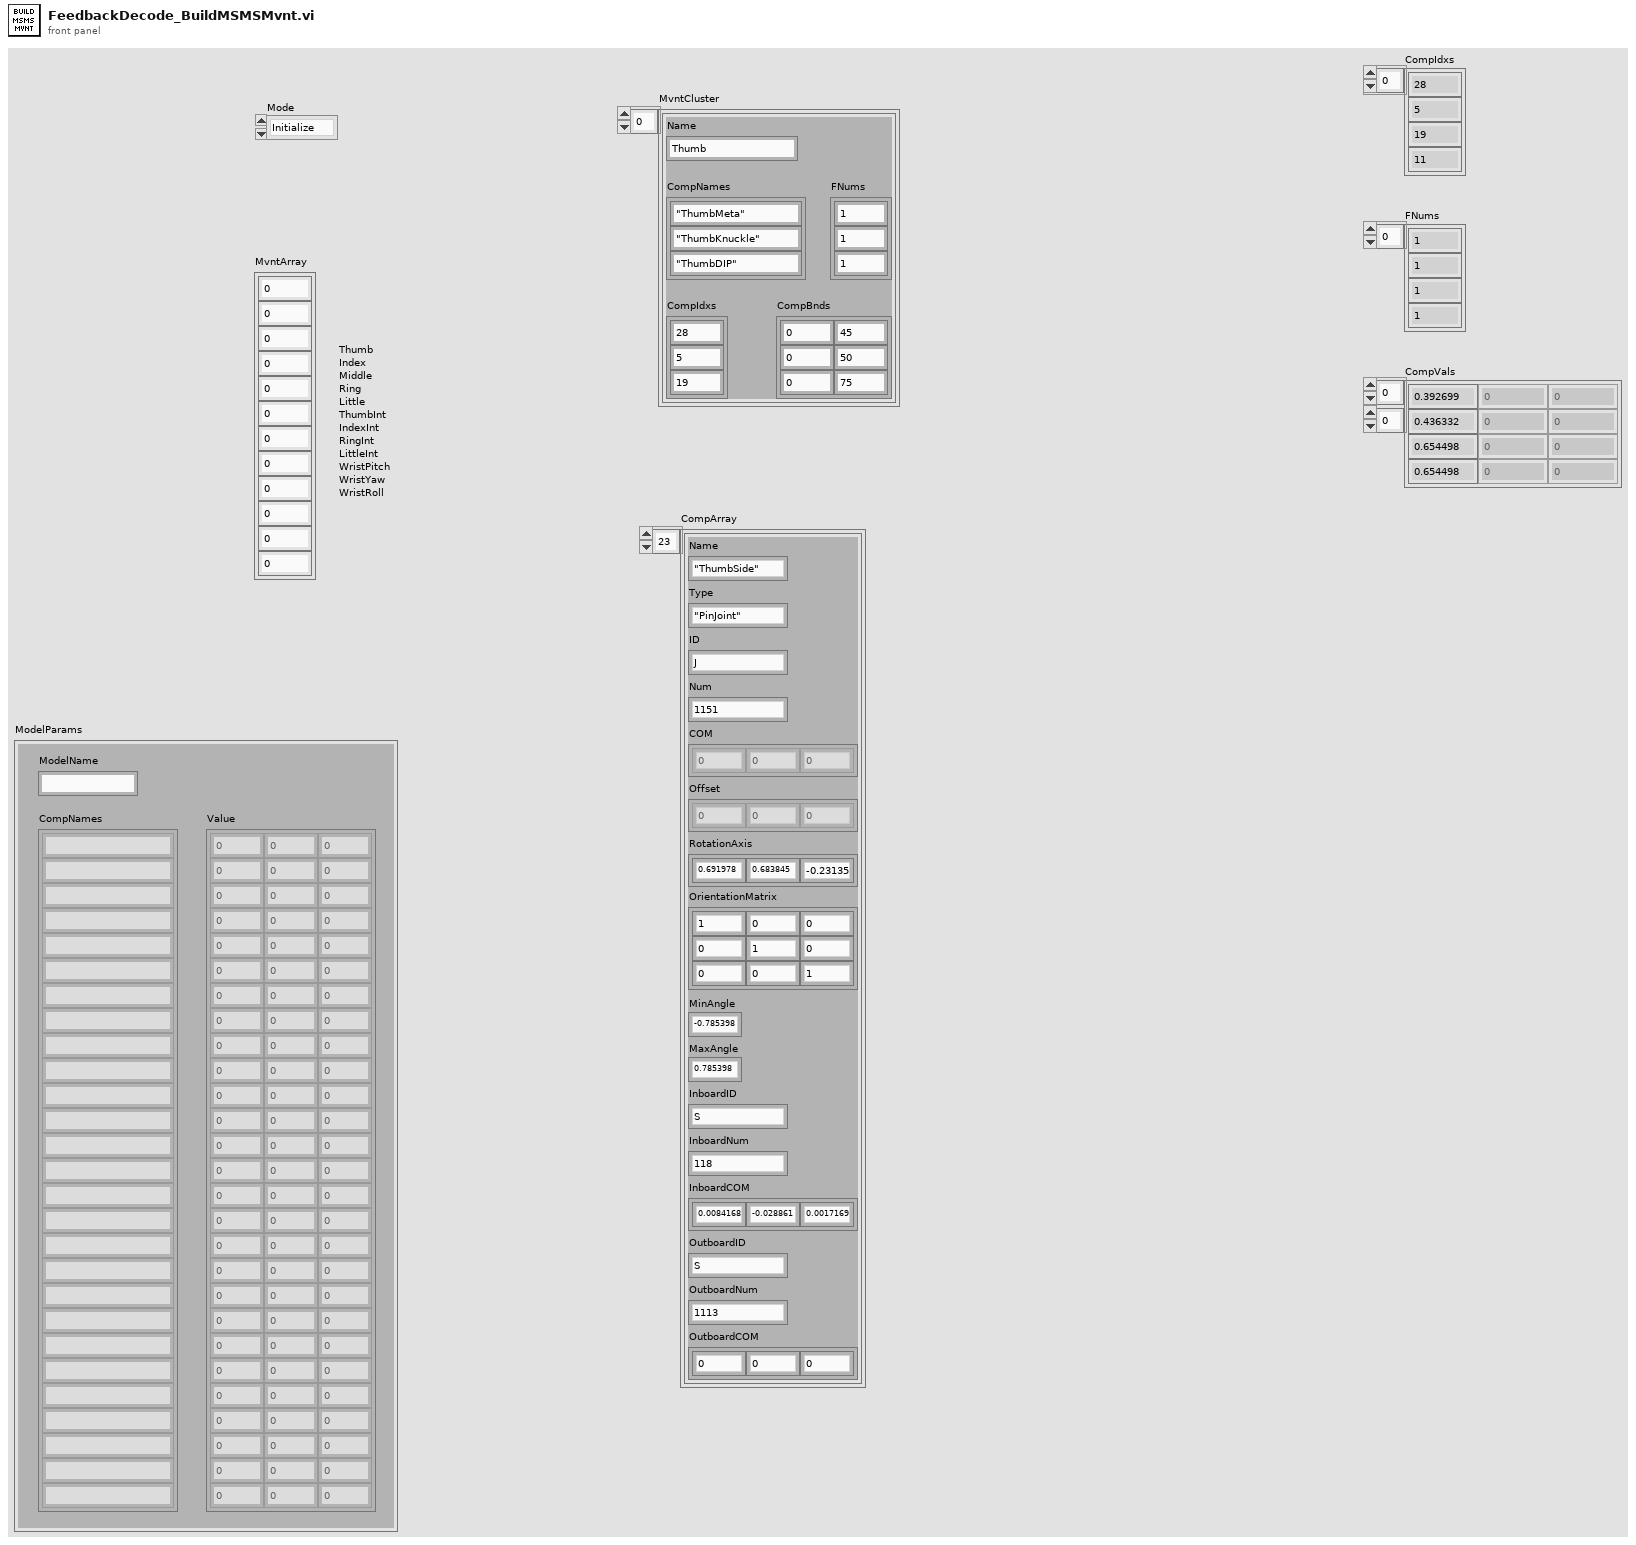
[diagram p1: front panel]
types:
  T1 = cluster{"ModelName":string, "Value":dbl[][], "CompNames":string[]}
  T2 = cluster{"Name":string, "Type":string, "ID":string, "Num":string, "COM":dbl[], "Offset":dbl[], "RotationAxis":dbl[], "OrientationMatrix":dbl[][], "MinAngle":dbl, "MaxAngle":dbl, "InboardID":string, "InboardNum":string, "InboardCOM":dbl[], "OutboardID":string, "OutboardNum":string, "OutboardCOM":dbl[]}[]
  T3 = cluster{"Name":string, "CompNames":string[], "FNums":i16[], "CompIdxs":i32[], "CompBnds":dbl[][]}[]
  T4 = cluster{"Name":string, "CompNames":string[], "FNums":i16[], "CompIdxs":i32[], "CompBnds":dbl[][]}
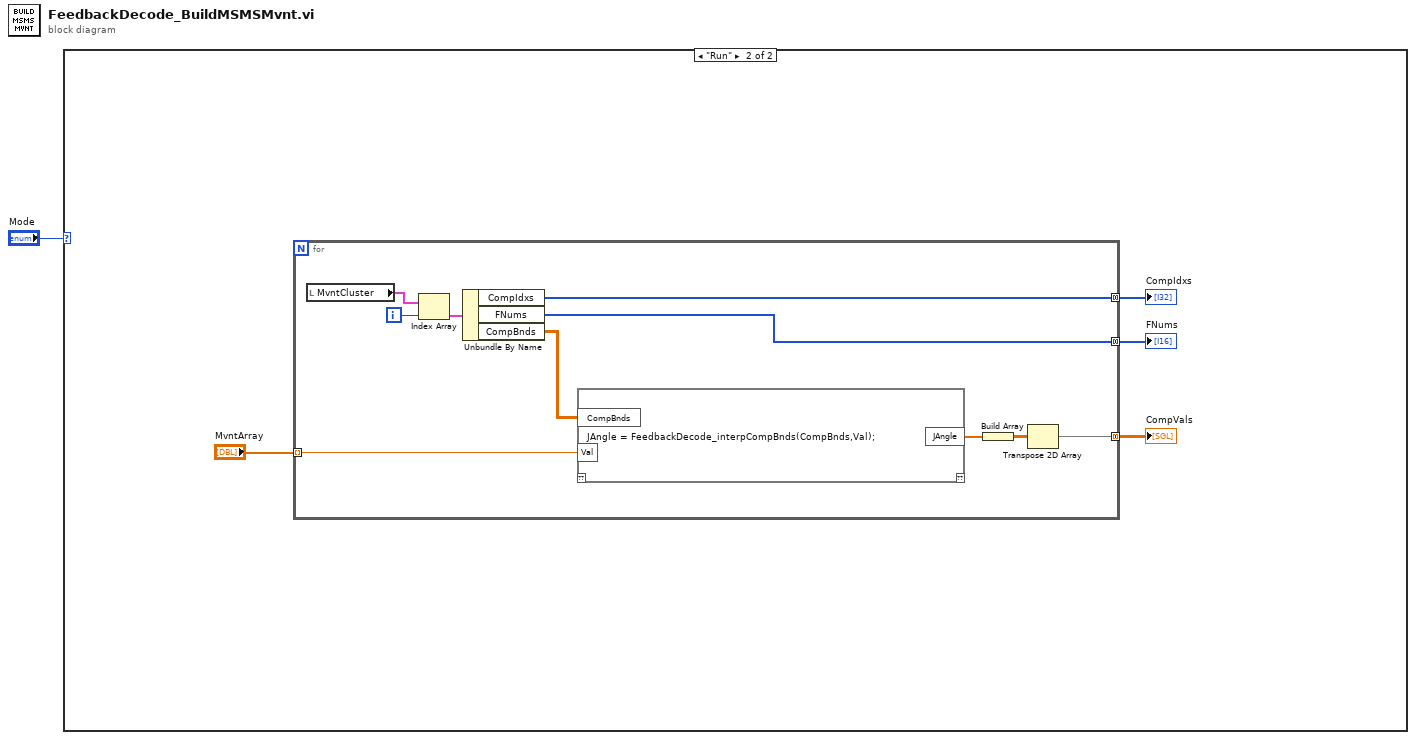
[diagram p0: block diagram]
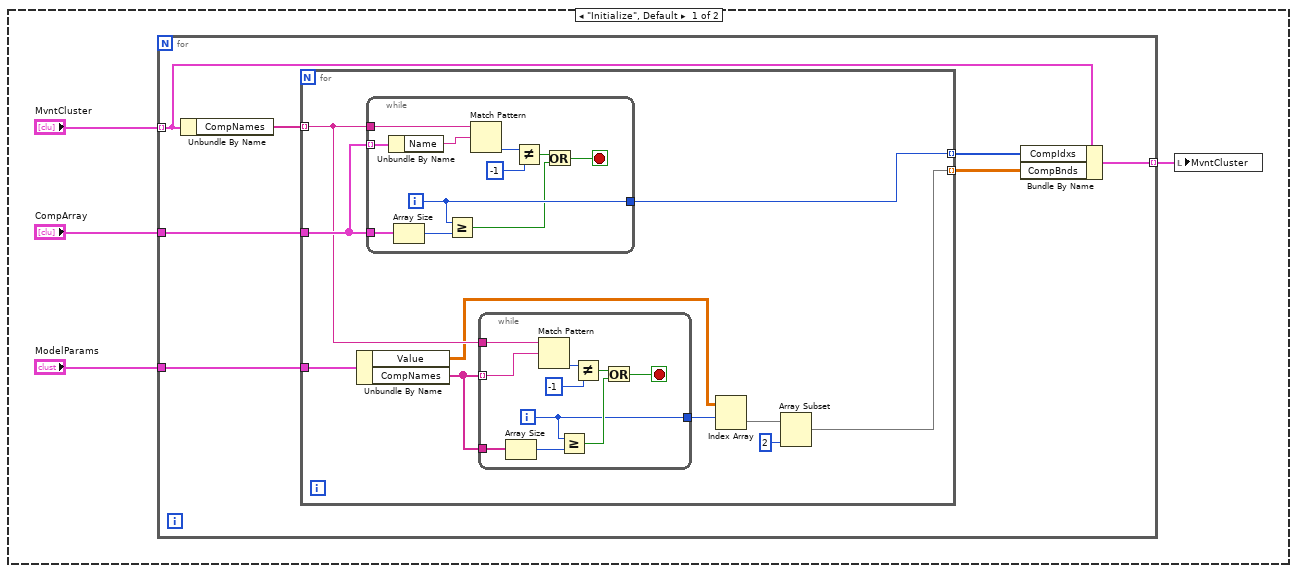
[diagram p2: hidden frame]
diagram:
  n1 = case shown="\"Run\"" "Mode" {
    frame "Initialize", Default {
      n2 = for {
        tunnel: "MvntCluster" -> [w10] mode=indexing
        tunnel: "CompArray" -> [w11]
        tunnel: [w8] -> w3 mode=indexing
        tunnel: "ModelParams" -> [w6]
        n3 = Unbundle By Name(w10) -> ("CompNames"=w12:string[])
        n4 = for {
          tunnel: w12 -> [w20] mode=indexing
          tunnel: [w22] -> w9 mode=indexing
          tunnel: w11 -> [w21]
          tunnel: [w13] -> w7 mode=indexing
          tunnel: w6 -> [w19]
          n5 = Unbundle By Name(w19) -> ("Value"=w16:dbl[][], "CompNames"=w18:string[])
          n6 = while {
            tunnel: w20 -> [w43]
            tunnel: w21 -> [w42] mode=indexing
            tunnel: [w37] -> w22
            tunnel: w21 -> [w33]
            i -> [w37]
            stop <- w34 stop-if-true
            n7 = Unbundle By Name(w42) -> ("Name"=w41:string)
            n8 = Array Size(array=w33) -> (size(s)=w38:i32)
            n9 = Greater Or Equal?(x=w37, y=w38) -> (x >= y?=w35:bool)
            n10 = Match Pattern(string=w43, regular expression=w41) -> (offset past match=w39:i32)  [unwired: 1 in, 3 out]
            n11 = Not Equal?(x=w39, y=-1) -> (x != y?=w36:bool)
            n12 = Or(x=w36, y=w35) -> (x .or. y?=w34:bool)
          }
          n13 = while {
            tunnel: w20 -> [w32]
            tunnel: w18 -> [w24]
            tunnel: w18 -> [w25] mode=indexing
            tunnel: [w23] -> w17
            i -> [w23]
            stop <- w26 stop-if-true
            n14 = Array Size(array=w24) -> (size(s)=w29:i32)
            n15 = Match Pattern(string=w32, regular expression=w25) -> (offset past match=w30:i32)  [unwired: 1 in, 3 out]
            n16 = Greater Or Equal?(x=w23, y=w29) -> (x >= y?=w27:bool)
            n17 = Not Equal?(x=w30, y=-1) -> (x != y?=w28:bool)
            n18 = Or(x=w28, y=w27) -> (x .or. y?=w26:bool)
          }
          n19 = Index Array(array=w16, index (row)=w17) -> (element=w15:dbl[])  [unwired: 1 in]
          n20 = Array Subset(array=w15, length=2) -> (w13:dbl[])  [unwired: 1 in]
        }
        n21 = Bundle By Name(cluster=w10, "CompIdxs"=w9, "CompBnds"=w7) -> (w8:T4)
      }
      n22 = local write "MvntCluster"(w3) -> ()
    }
    frame "Run" {
      n23 = for {
        tunnel: [w55] -> w47 mode=concatenating
        tunnel: [w54] -> w46 mode=concatenating
        tunnel: [w51] -> w45 mode=concatenating
        tunnel: "MvntArray" -> [w49] mode=indexing
        i -> [w50]
        n24 = local read "MvntCluster"() -> (w48:T3)
        n25 = Index Array(array=w48, index=w50) -> (element=w57:T4)
        n26 = Unbundle By Name(w57) -> ("CompIdxs"=w55:i32[], "FNums"=w54:i16[], "CompBnds"=w56:dbl[][])
        n27 = mathscript code="JAngle = FeedbackDecode_interpCompBnds(CompBnds,Val);"("CompBnds"=w56, "Val"=w49) -> ("JAngle"=w53:dbl[])  [unwired: 1 in, 1 out]
        n28 = Build Array(w53) -> (w52:dbl[][])
        n29 = Transpose 2D Array(2D array=w52) -> (transposed array=w51:dbl[][])
      }
      "CompVals" <- w45
      "CompIdxs" <- w47
      "FNums" <- w46
    }
  }
